vi "MyrioProject.vi"() -> ()   [LabVIEW 2018]
doc: "The myRIO Project template acquires acceleration data from the onboard accelerometer and displays the changes of acceleration values in a waveform chart."
uses:
  <vilib>/myRIO/Common/Instrument Driver Framework/myRIO v1.0/Encoder/typedefs/Encoder Signal Mode.ctl
  <vilib>/Platform/TimedLoop/XDataNode/timing_clust.ctl
  <vilib>/Platform/TimedLoop/XDataNode/nitl_modes.ctl
  <vilib>/Platform/TimedLoop/XDataNode/wakeup.ctl
  <vilib>/Analysis/Matrix/Datatypes/RealMatrix.ctl
  <vilib>/myRIO/Instrument Drivers/Onboard IO/PWM/typedefs/PWM Reference.ctl
  <vilib>/myRIO/Common/Instrument Driver Framework/Utilities/typedefs/myRIO Generic Hardware Reference.ctl
  <vilib>/myRIO/Common/Instrument Driver Framework/Utilities/typedefs/Hardware Version Enum.ctl
  <vilib>/myRIO/Common/Instrument Driver Framework/Utilities/typedefs/myRIO v1.0 Reference.ctl
  <vilib>/myRIO/Common/Instrument Driver Framework/Utilities/typedefs/Generic FPGA Reference.ctl
  <vilib>/myRIO/Common/Instrument Driver Framework/myRIO v1.0/PWM/typedefs/PWM Channels Enum.ctl
  <vilib>/myRIO/Instrument Drivers/Onboard IO/PWM/typedefs/PWM Configuration.ctl
  <vilib>/userdefined/High Color/nirio_resource_hc.ctl
  <vilib>/myRIO/Common/Instrument Driver Framework/myRIO v1.0/Encoder/typedefs/Encoder Configuration v1.0.ctl
  <vilib>/myRIO/Instrument Drivers/Onboard IO/Encoder/typedefs/Encoder Reference.ctl
  <vilib>/myRIO/Common/Instrument Driver Framework/myRIO v1.0/Encoder/typedefs/Encoder Channels Enum.ctl
  <vilib>/myRIO/Instrument Drivers/Onboard IO/DIO/typedefs/DIO Reference.ctl
  <vilib>/myRIO/Common/Instrument Driver Framework/myRIO v1.0/DIO/typedefs/DIO Channels List.ctl
  <vilib>/myRIO/Common/Instrument Driver Framework/myRIO v1.0/DIO/typedefs/DIO Channels Enum.ctl
  <vilib>/myRIO/Instrument Drivers/Onboard IO/AI/typedefs/AI Reference.ctl
  <vilib>/myRIO/Common/Instrument Driver Framework/myRIO v1.0/AI/typedefs/AI Channels List.ctl
  <vilib>/myRIO/Common/Instrument Driver Framework/myRIO v1.0/AI/typedefs/AI Channels Enum.ctl
  <vilib>/myRIO/Common/Instrument Driver Framework/Utilities/typedefs/Analog Scaling Constants List.ctl
  <vilib>/myRIO/Common/Instrument Driver Framework/Utilities/typedefs/Analog Scaling Constants.ctl
  <vilib>/myRIO/Common/Instrument Driver Framework/myRIO v1.0/PWM/vis/myRIO v1.1 Open PWM.vi
  <vilib>/myRIO/Common/Instrument Driver Framework/myRIO v1.0/Encoder/vis/myRIO v1.1 Open Encoder.vi
  <vilib>/myRIO/Common/Instrument Driver Framework/Utilities/vis/Is FPGA Ref Available.vi
  <vilib>/myRIO/Common/Instrument Driver Framework/myRIO v1.0/AI/vis/myRIO v1.1 Open AI.vi
  <vilib>/myRIO/Common/Instrument Driver Framework/myRIO v1.0/DIO/vis/myRIO v1.1 Open DIO.vi
  <vilib>/myRIO/Instrument Drivers/Onboard IO/PWM/vis/Set Duty Cycle and Frequency.vi
  <vilib>/myRIO/Instrument Drivers/Onboard IO/DIO/vis/Write.vi
  <vilib>/myRIO/Common/Instrument Driver Framework/Utilities/vis/Validate Channels.vi
  <vilib>/myRIO/Common/Instrument Driver Framework/myRIO v1.0/PWM/vis/myRIO v1.0 Reserve PWM.vi
  <vilib>/myRIO/Common/Instrument Driver Framework/myRIO v1.0/Encoder/vis/myRIO v1.0 Reserve Encoder.vi
  <vilib>/myRIO/Common/Instrument Driver Framework/myRIO v1.0/AI/vis/myRIO v1.0 Reserve AI.vi
  <vilib>/myRIO/Common/Instrument Driver Framework/myRIO v1.0/DIO/vis/myRIO v1.0 Reserve DIO.vi
  <vilib>/myRIO/Common/Instrument Driver Framework/myRIO v1.0/Encoder/vis/myRIO v1.0 Close Encoder.vi
  <vilib>/myRIO/Common/Instrument Driver Framework/myRIO v1.0/PWM/vis/myRIO v1.0 Close PWM.vi
  <vilib>/myRIO/Common/Instrument Driver Framework/myRIO v1.0/PWM/vis/myRIO v1.0 Build MUX Configuration PWM.vi
  <vilib>/myRIO/Common/Instrument Driver Framework/myRIO v1.0/Resource Manager/vis/myRIO v1.0 Reserve Channel List.vi
  <vilib>/myRIO/Common/Instrument Driver Framework/myRIO v1.0/Encoder/vis/myRIO v1.0 Build MUX Configuration Encoder.vi
  <vilib>/myRIO/Common/Instrument Driver Framework/myRIO v1.0/AI/vis/myRIO v1.0 Build MUX Configuration AI.vi
  <vilib>/myRIO/Common/Instrument Driver Framework/myRIO v1.0/DIO/vis/myRIO v1.0 Build MUX Configuration DIO.vi
  <vilib>/myRIO/Common/Instrument Driver Framework/myRIO v1.0/Encoder/vis/myRIO v1.0 Unreserve Encoder.vi
  <vilib>/myRIO/Common/Instrument Driver Framework/myRIO v1.0/PWM/vis/myRIO v1.0 Unreserve PWM.vi
  <vilib>/myRIO/Common/Instrument Driver Framework/myRIO v1.0/Resource Manager/vis/myRIO v1.0 Create Configuration List.vi
  <vilib>/myRIO/Common/Instrument Driver Framework/myRIO v1.0/Resource Manager/vis/myRIO v1.0 Reserve Channel.vi
  <vilib>/myRIO/Common/Instrument Driver Framework/myRIO v1.0/Resource Manager/vis/myRIO v1.0 Unreserve Channel.vi
  <vilib>/myRIO/Common/Instrument Driver Framework/myRIO v1.0/Resource Manager/vis/myRIO v1.0 Unreserve Channel List.vi
  <vilib>/myRIO/Common/Instrument Driver Framework/myRIO v1.0/Resource Manager/vis/myRIO v1.0 Build Mutex Name.vi
  <vilib>/Utility/VariantDataType/GetNumericInfo.vi
  <vilib>/Utility/error.llb/Error Cluster From Error Code.vi
  <vilib>/myRIO/Common/Instrument Driver Framework/myRIO v1.0/myRIO v1.1 Open.vi
  <vilib>/myRIO/Common/Instrument Driver Framework/Utilities/vis/IO Manager.vi
  <vilib>/myRIO/Common/Instrument Driver Framework/Utilities/vis/Configuration Manager.vi
  <vilib>/myRIO/Common/Instrument Driver Framework/myRIO v1.0/Resource Manager/vis/myRIO v1.0 Configure IO.vi
  <vilib>/myRIO/Common/Instrument Driver Framework/myRIO v1.0/myRIO v1.0 Close.vi
  <vilib>/myRIO/Common/Instrument Driver Framework/myRIO v1.0/PWM/vis/myRIO v1.0 Write PWM.vi
  <vilib>/myRIO/Common/Instrument Driver Framework/myRIO v1.0/Encoder/vis/myRIO v1.0 Configure Encoder.vi
  <vilib>/myRIO/Common/Instrument Driver Framework/myRIO v1.0/Encoder/vis/myRIO v1.0 Enable Encoder.vi
  <vilib>/myRIO/Common/Instrument Driver Framework/myRIO v1.0/DIO/vis/myRIO v1.0 Read DIO.vi
  <vilib>/myRIO/Common/Instrument Driver Framework/myRIO v1.0/AI/vis/myRIO v1.0 Get Scaling Constants AI.vi
  <vilib>/myRIO/Common/Instrument Driver Framework/myRIO v1.0/AI/vis/myRIO v1.0 Read AI.vi
  <vilib>/myRIO/Common/Instrument Driver Framework/myRIO v1.0/Encoder/vis/myRIO v1.0 Read Encoder.vi
  <vilib>/myRIO/Common/Instrument Driver Framework/myRIO v1.0/DIO/vis/myRIO v1.0 Write DIO.vi
  <vilib>/myRIO/Common/Instrument Driver Framework/myRIO v1.0/Encoder/vis/myRIO v1.0 Shutdown Encoder.vi
  <vilib>/myRIO/Common/Instrument Driver Framework/myRIO v1.0/PWM/vis/myRIO v1.0 Shutdown PWM.vi
  <vilib>/platform/TimedLoop/XDataNode/XDataNode.xnode
  <vilib>/myRIO/Instrument Drivers/Onboard IO/PWM/vis/myRIO PWM Open.xnode
  <vilib>/myRIO/Instrument Drivers/Onboard IO/Encoder/vis/myRIO Encoder Open.xnode
  <vilib>/myRIO/Express VI/Onboard IO/PWM/PWM Express VI.xnode
  <vilib>/myRIO/Express VI/Onboard Devices/Button/Button Express VI.xnode
  <vilib>/myRIO/Instrument Drivers/Onboard IO/DIO/vis/myRIO DIO Open.xnode
  <vilib>/myRIO/Express VI/Onboard IO/AI/AI Express VI.xnode
  <vilib>/myRIO/Instrument Drivers/Onboard IO/AI/vis/myRIO AI Open.xnode
  <vilib>/myRIO/Express VI/Onboard IO/DO/DO Express VI.xnode
  <vilib>/myRIO/Instrument Drivers/Onboard IO/Encoder/Encoder.lvlib
  <vilib>/myRIO/Instrument Drivers/Onboard IO/PWM/PWM.lvlib
  <vilib>/myRIO/Instrument Drivers/Onboard IO/DIO/DIO.lvlib
  <vilib>/myRIO/Instrument Drivers/Onboard IO/AI/AI.lvlib
  <vilib>/Platform/TimedLoop/XDataNode/XDNodeRunTimeDep.lvlib
  <vilib>/Analysis/Matrix/NI_Matrix.lvlib
panel:
  in  "Start":bool
  in  "Stop Button":bool
  out "element":dbl
  out "element 2":dbl
  in  "manual":bool
  out "Numeric Control":dbl
  out "data":dbl
  out "sensor2 (A/AI2 (Pin 7))":dbl
  out "sensor1":dbl
  out "stallRojo (A/AI0 (Pin 3))":dbl
  out "stallBlanco (A/AI1 (Pin 5))":dbl
  out "subarray 2":dbl[][](array[numeric])
  out "subarray":dbl[][](array[numeric])
  out "vectores":dbl[][][](array[numeric])
  in  "saturacion":dbl=0.3
  in  "Duty Cycle 2":dbl(slide)=0.5 scale=0.05..0.1
  in  "Duty Cycle":dbl(slide)=0.5 scale=0.05..0.1
  in  "Reset Counter 2":bool
  in  "Reset Counter":bool
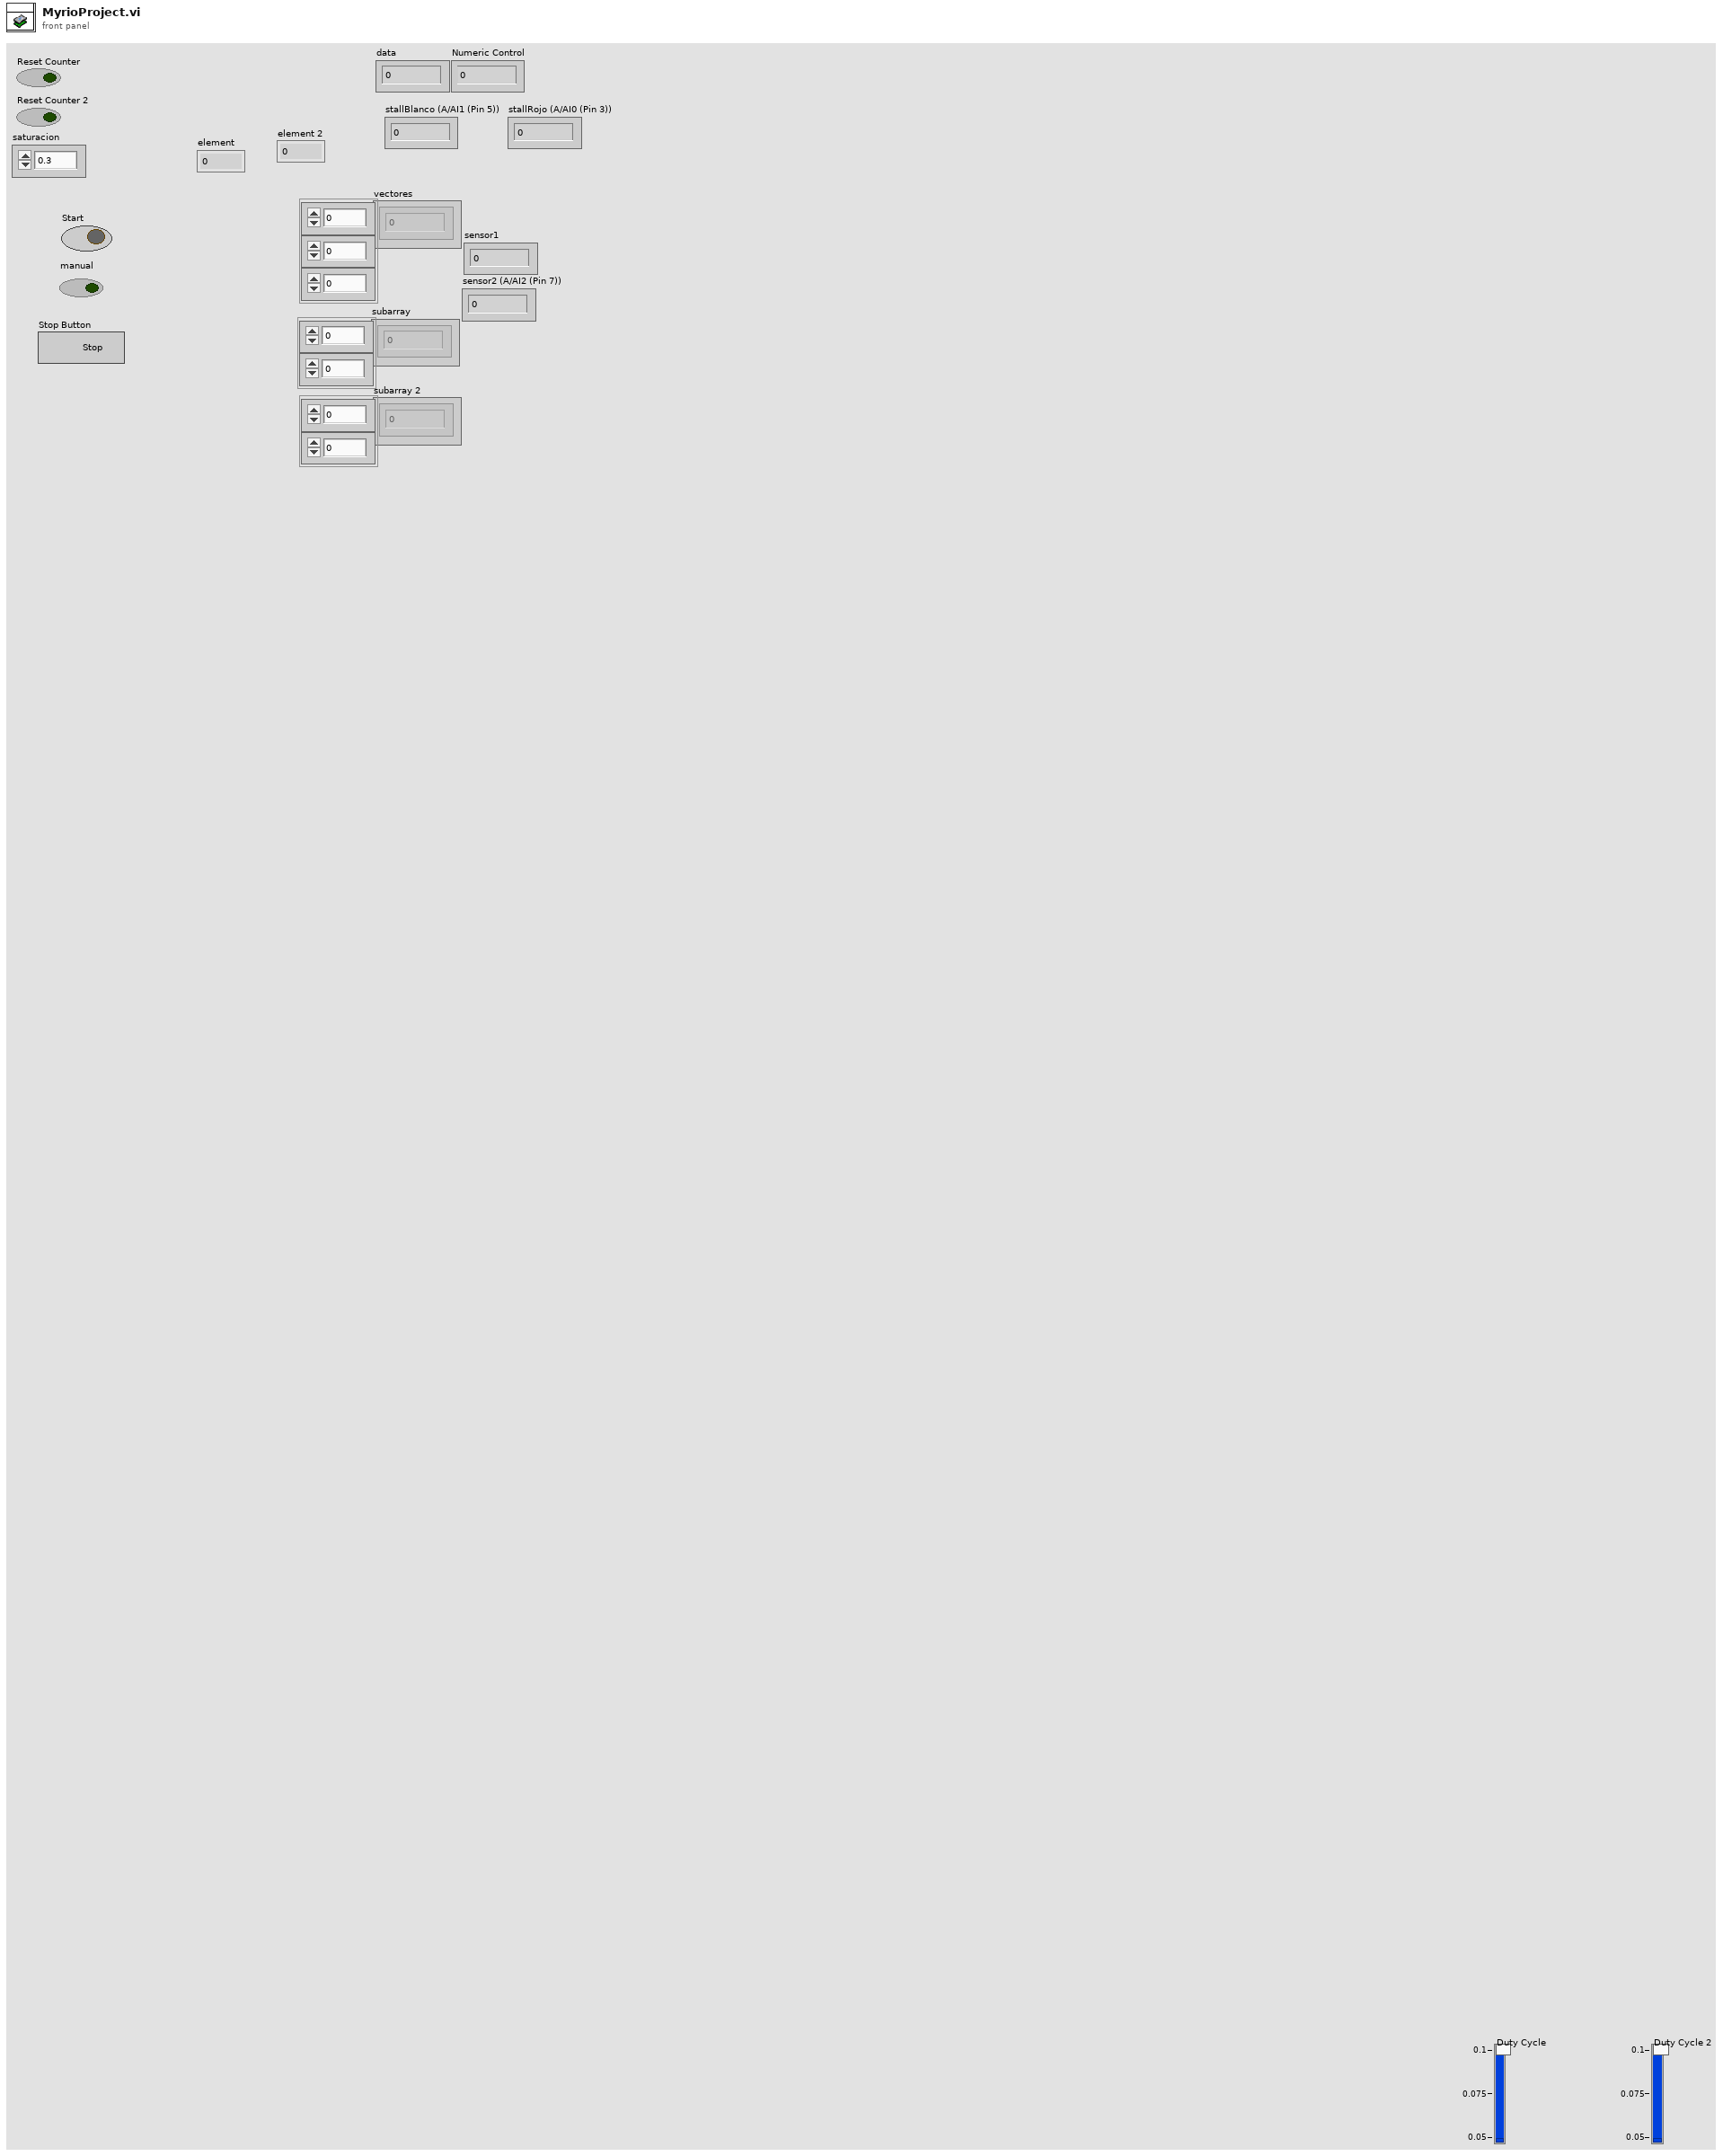
[diagram p1: front panel]
types:
  T1 = typedef "NI_Matrix.lvlib/RealMatrix.ctl" = dbl[][]
  T2 = enum16{"normal", "grande-Sensor", "grande home", "peque-sensor", "peque- home", "peque-reset"}
  T3 = typedef "Encoder Signal Mode.ctl" = enum16{"Quadrature phase signal", "Step and direction signal"}
  T4 = typedef "PWM.lvlib/PWM Reference.ctl" = cluster{"myRIO Reference":T5, "PWM Channels Enum":T9, "PWM Configuration":T10}
  T5 = typedef "myRIO Generic Hardware Reference.ctl" = cluster{"myRIO Model":T6, "myRIO Hardware Reference":T7}
  T6 = typedef "Hardware Version Enum.ctl" = enum16{"Unknown", "myRIO-1900", "myRIO-1950", "roboRIO", "NI ELVIS RIO CM", "ELVIS III"}
  T7 = typedef "myRIO v1.0 Reference.ctl" = cluster{"Generic FPGA Reference":T8, "Allow multiple opens":bool}
  T8 = typedef "Generic FPGA Reference.ctl" = refnum<k20>
  T9 = typedef "PWM Channels Enum.ctl" = enum16{"Not Connected", "C/PWM0", "C/PWM1", "A/PWM0", "A/PWM1", "A/PWM2", "A/PWM3", "A/PWM4", "A/PWM5", "A/PWM6", "A/PWM7", "A/PWM8", "A/PWM9", "A/PWM10", "A/PWM11", "A/PWM12", "A/PWM13", "A/PWM14", "A/PWM15", "A/PWM16", "A/PWM17", "A/PWM18", "A/PWM19", "B/PWM0", "B/PWM1", "B/PWM2", "B/PWM3", "B/PWM4", "B/PWM5", "B/PWM6", "B/PWM7", "B/PWM8", "B/PWM9", "B/PWM10", "B/PWM11", "B/PWM12", "B/PWM13", "B/PWM14", "B/PWM15", "B/PWM16", "B/PWM17", "B/PWM18", "B/PWM19", "PWM/PWM0", "PWM/PWM1", "PWM/PWM2", "PWM/PWM3", "PWM/PWM4", "PWM/PWM5", "PWM/PWM6", "PWM/PWM7", "PWM/PWM8", "PWM/PWM9"}
  T10 = typedef "PWM.lvlib/PWM Configuration.ctl" = cluster{"Frequency":dbl, "Duty Cycle":dbl}
  T11 = typedef "Encoder.lvlib/Encoder Reference.ctl" = cluster{"myRIO Reference":T5, "Encoder Channels Enum":T12}
  T12 = typedef "Encoder Channels Enum.ctl" = enum16{"Not Connected", "C/ENC0", "C/ENC1", "A/ENC", "A/ENC0", "A/ENC1", "A/ENC2", "A/ENC3", "A/ENC4", "A/ENC5", "A/ENC6", "A/ENC7", "A/ENC8", "A/ENC9", "B/ENC", "B/ENC0", "B/ENC1", "B/ENC2", "B/ENC3", "B/ENC4", "B/ENC5", "B/ENC6", "B/ENC7", "B/ENC8", "B/ENC9", "DIO/ENC0", "DIO/ENC1", "DIO/ENC2", "DIO/ENC3", "DIO/ENC4"}
  T13 = cluster{"Double":dbl, "dbl Scaled Value":dbl, "Output":dbl, "seconds since 1Jan1904":timestamp, dbl, dbl, dbl}
  T14 = typedef "XDNodeRunTimeDep.lvlib/timing_clust.ctl" = cluster{"Expected End [f-1]":u64, "Actual End [f-1]":u64, "Finished Late? [f-1]":bool, "Expected End [i-1]":u64, "Actual End [i-1]":u64, "Finished Late? [i-1]":bool, "Expected Start [i]":u64, "Actual Start [i]":u64, "Expected Start [f]":u64, "Actual Start [f]":u64, "Source Name":string, "Structure Name":string, "Period":i64, "Deadline":i64, "Offset":i64, "Start":i64, "Priority":i32, "Timeout":i32, "Mode":T15, "Wakeup Reason":T16, "Error":errorcluster, "Source Type":string, "Secondary Source Type":string, "Global End Time":u64, "Global Start Time":u64, "Frame Duration":u64, "Iteration Duration":u64, "Assigned CPU":i32, "I/O Scan Engine Mode":u32}
  T15 = typedef "XDNodeRunTimeDep.lvlib/nitl_modes.ctl" = enum32{"No Change", "Process missed periods, maintain original phase", "Discard missed periods, maintain original phase", "Process missed periods, ignore original phase", "Discard missed periods, ignore original phase"}
  T16 = typedef "XDNodeRunTimeDep.lvlib/wakeup.ctl" = enum32{"Normal", "Aborted", "Asynchronous wakeup", "Timing source error", "Timed loop error", "Timeout"}
  T17 = typedef "nirio_resource_hc.ctl" = tag
  T18 = typedef "AI.lvlib/AI Reference.ctl" = cluster{"myRIO Reference":T5, "AI Channels List":T19, "AI Scaling Constants List":T21}
  T19 = typedef "AI Channels List.ctl" = T20[]
  T20 = typedef "AI Channels Enum.ctl" = enum16{"Not Connected", "AudioIn/Left", "AudioIn/Right", "C/AI0", "C/AI1", "A/AI0", "A/AI1", "A/AI2", "A/AI3", "A/AI4", "A/AI5", "A/AI6", "A/AI7", "B/AI0", "B/AI1", "B/AI2", "B/AI3", "B/AI4", "B/AI5", "B/AI6", "B/AI7", "AI/AI0", "AI/AI1", "AI/AI2", "AI/AI3", "A/AI0 (DIFF)", "A/AI1 (DIFF)", "A/AI2 (DIFF)", "A/AI3 (DIFF)", "B/AI0 (DIFF)", "B/AI1 (DIFF)", "B/AI2 (DIFF)", "B/AI3 (DIFF)"}
  T21 = typedef "Analog Scaling Constants List.ctl" = T22[]
  T22 = typedef "Analog Scaling Constants.ctl" = cluster{"LSB Weight (Volts)":dbl, "Offset (Volts)":dbl, "Signed?":bool}
  T23 = typedef "DIO.lvlib/DIO Reference.ctl" = cluster{"myRIO Reference":T5, "DIO Channels List":T24}
  T24 = typedef "DIO Channels List.ctl" = T25[]
  T25 = typedef "DIO Channels Enum.ctl" = enum16{"Not Connected", "C/DIO0", "C/DIO1", "C/DIO2", "C/DIO3", "C/DIO4", "C/DIO5", "C/DIO6", "C/DIO7", "A/DIO0", "A/DIO1", "A/DIO2", "A/DIO3", "A/DIO4", "A/DIO5", "A/DIO6", "A/DIO7", "A/DIO8", "A/DIO9", "A/DIO10", "A/DIO11", "A/DIO12", "A/DIO13", "A/DIO14", "A/DIO15", "A/DIO16", "A/DIO17", "A/DIO18", "A/DIO19", "B/DIO0", "B/DIO1", "B/DIO2", "B/DIO3", "B/DIO4", "B/DIO5", "B/DIO6", "B/DIO7", "B/DIO8", "B/DIO9", "B/DIO10", "B/DIO11", "B/DIO12", "B/DIO13", "B/DIO14", "B/DIO15", "B/DIO16", "B/DIO17", "B/DIO18", "B/DIO19", "LED0", "LED1", "LED2", "LED3", "Button0", "DIO/DIO0", "DIO/DIO1", "DIO/DIO2", "DIO/DIO3", "DIO/DIO4", "DIO/DIO5", "DIO/DIO6", "DIO/DIO7", "DIO/DIO8", "DIO/DIO9", "SPI/CS0", "SPI/CS1", "SPI/CS2", "SPI/CS3", "LED RADIO (Green)", "LED RADIO (Red)", "LED COMM (Green)", "LED COMM (Red)", "LED MODE (Green)", "LED MODE (Red)"}
  T26 = cluster{dbl, dbl, "Counter Value":i32, "seconds since 1Jan1904":timestamp, dbl, dbl, "Counter Value":i32}
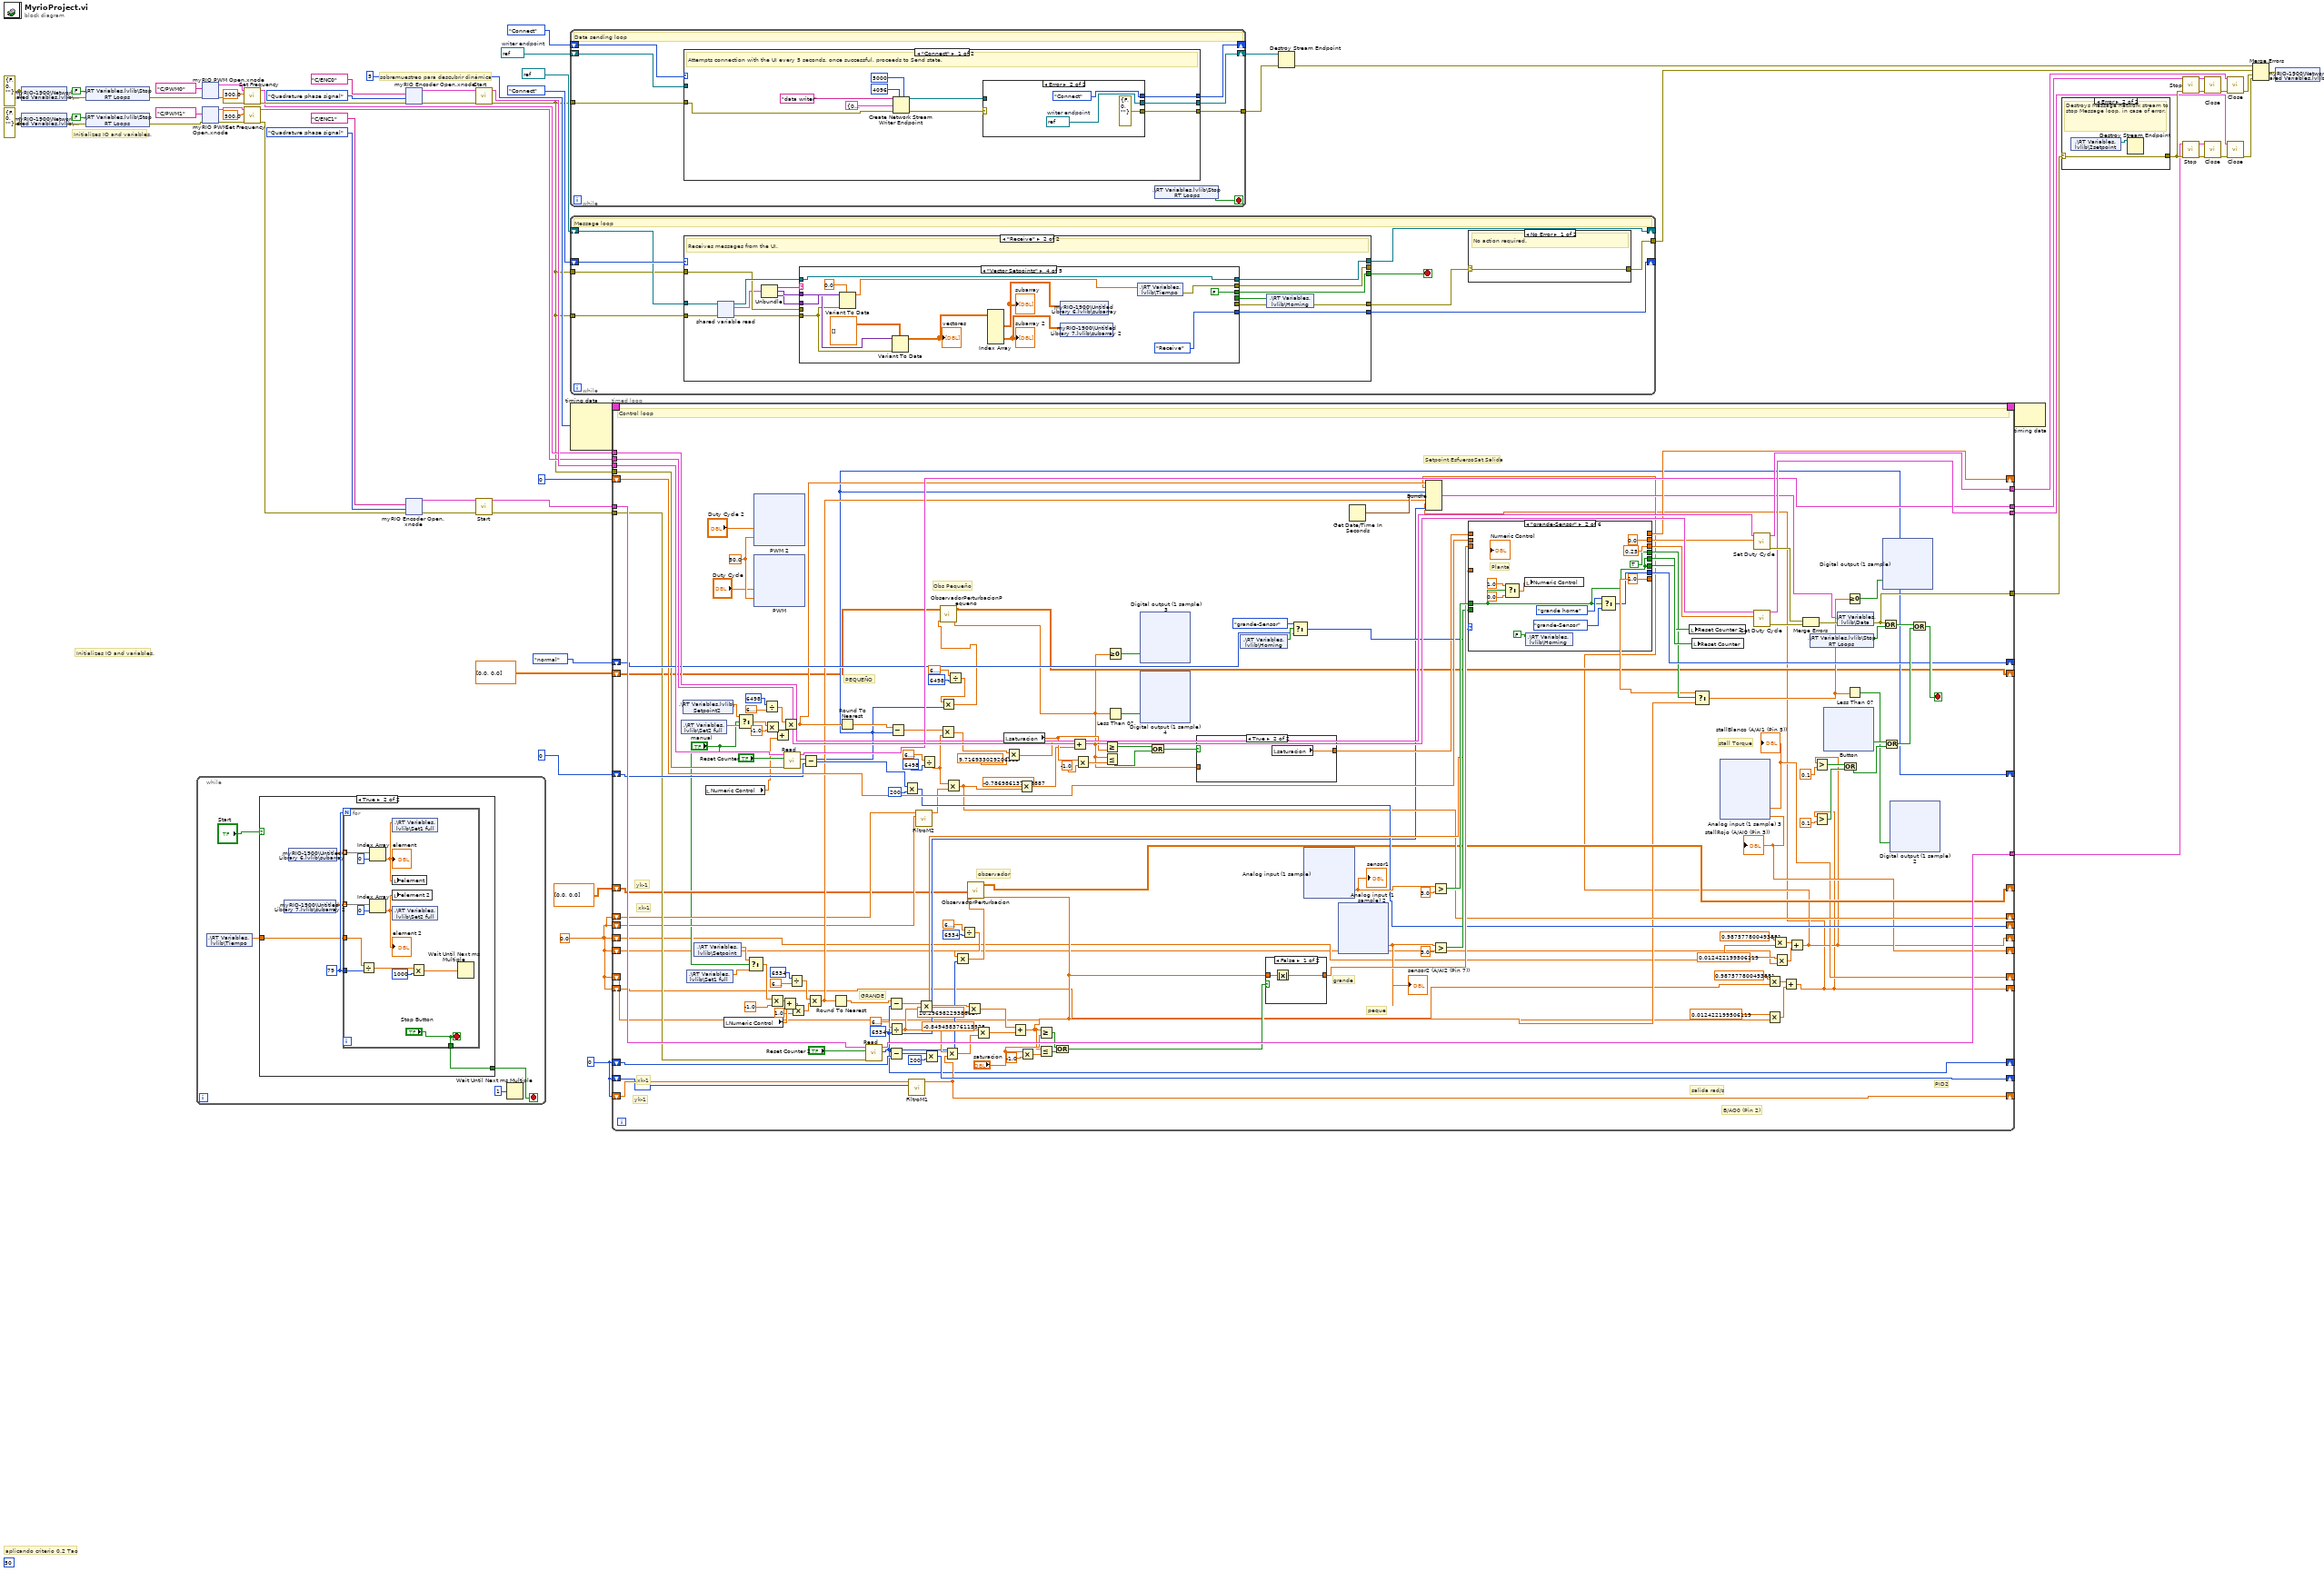
[diagram p0: block diagram]
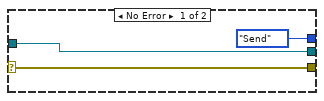
[diagram p4: hidden frame]
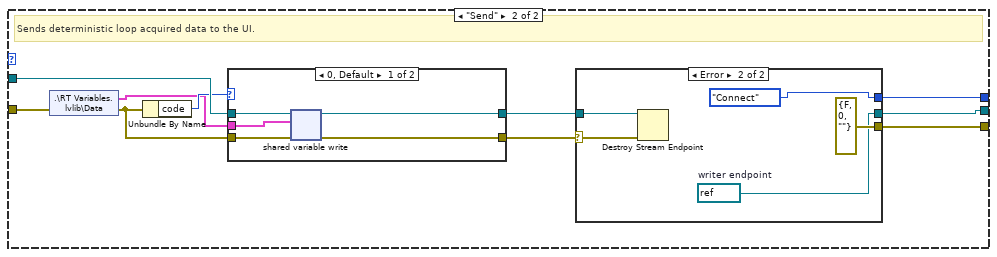
[diagram p5: hidden frame]
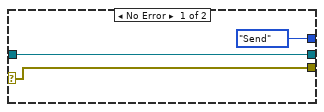
[diagram p6: hidden frame]
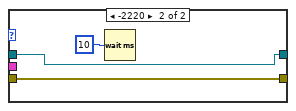
[diagram p7: hidden frame]
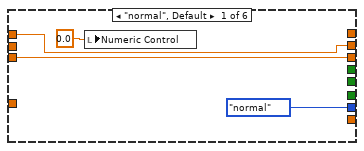
[diagram p8: hidden frame]
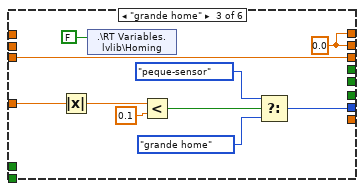
[diagram p9: hidden frame]
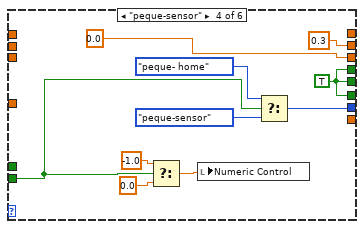
[diagram p10: hidden frame]
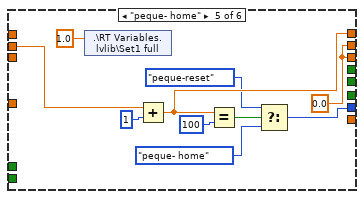
[diagram p11: hidden frame]
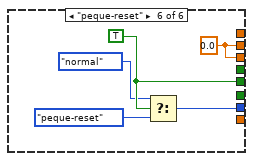
[diagram p12: hidden frame]
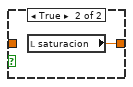
[diagram p13: hidden frame]
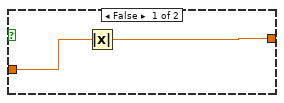
[diagram p14: hidden frame]
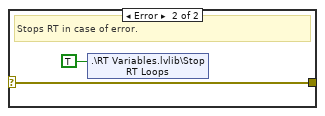
[diagram p15: hidden frame]
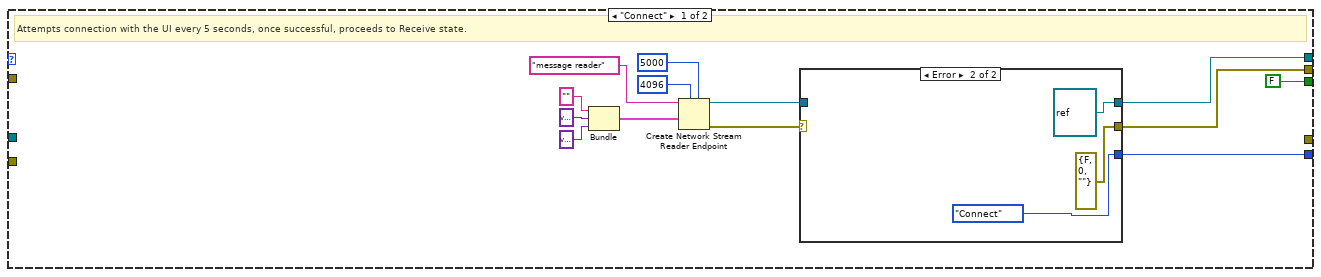
[diagram p16: hidden frame]
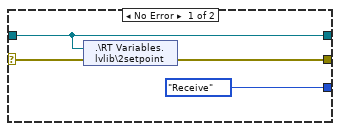
[diagram p17: hidden frame]
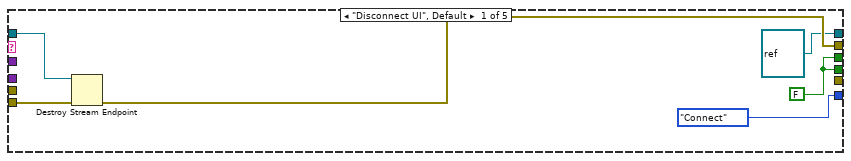
[diagram p18: hidden frame]
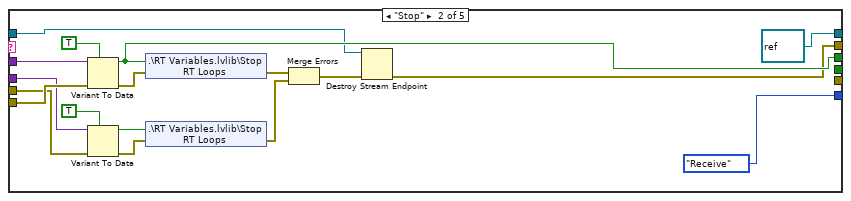
[diagram p19: hidden frame]
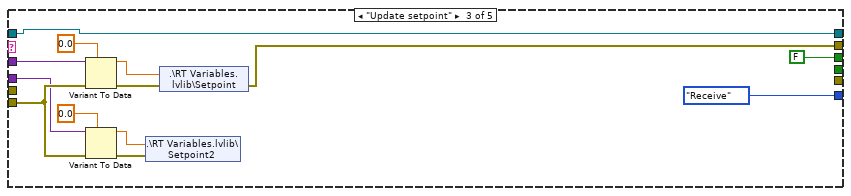
[diagram p20: hidden frame]
diagram:
  w1 = 0.0
  w2 = 0 ("Counter Value")
  (unwired) 50
  w19 = refnum<k21> refnum  # writer endpoint
  w32 = errorcluster {"status"=FALSE, "code"=0, "source"=""} ("error IO")
  w54 = errorcluster {"status"=FALSE, "code"=0, "source"=""} ("error IO")
  # "aplicando criterio 0.2 Tao"
  # "sobremuestreo para descubrir dinámica"
  # "Initializes IO and variables."
  # "Initializes IO and variables."
  n1 = shared-variable "myRIO-1900\\Network Shared Variables.lvlib\\error IO"(w54, error in=w54) -> (error out=w55:errorcluster)
  n2 = shared-variable "myRIO-1900\\Network Shared Variables.lvlib\\error IO"(w32, error in=w32) -> (error out=w33:errorcluster)
  n3 = shared-variable ".\\RT Variables.lvlib\\Stop RT Loops"(FALSE ("Stop RT Loops"), error in=w55) -> (error out=w42:errorcluster)
  n4 = shared-variable ".\\RT Variables.lvlib\\Stop RT Loops"(FALSE ("Stop RT Loops"), error in=w33) -> (error out=w25:errorcluster)
  n5 = while {
    stop <- w66 stop-if-true
    n6 = shared-variable ".\\RT Variables.lvlib\\Tiempo"() -> (w68:dbl)  [unwired: 1 in, 1 out]
    n7 = case shown="True" "Start" {
      tunnel: w68 -> [_ w71]
      tunnel: [_ w70] -> w66
      frame False {
      }
      frame True {
        w74 = 79
        n8 = shared-variable "myRIO-1900\\Untitled Library 7.lvlib\\subarray 2"() -> (w72:dbl[][])  [unwired: 1 in, 1 out]
        n9 = shared-variable "myRIO-1900\\Untitled Library 6.lvlib\\subarray"() -> (w73:dbl[][])  [unwired: 1 in, 1 out]
        n10 = for {
          N: w74 -> [_]
          tunnel: w74 -> [w84]
          tunnel: w73 -> [w83] mode=indexing
          tunnel: w72 -> [w80] mode=indexing
          tunnel: w71 -> [w76]
          tunnel: ["Stop Button"] -> w70
          stop <- "Stop Button" stop-if-true
          n11 = Divide(x=w76, y=w84) -> (x/y=w86:dbl)
          n12 = Index Array(array=w83, index=0) -> (element=w78:dbl)
          "element" <- w78
          n13 = Index Array(array=w80, index=0) -> (element=w77:dbl)
          "element 2" <- w77
          n14 = shared-variable ".\\RT Variables.lvlib\\Set1 full"(w78) -> ()  [unwired: 1 in, 1 out]
          n15 = local write "element"(w78) -> ()
          n16 = local write "element 2"(w77) -> ()
          n17 = shared-variable ".\\RT Variables.lvlib\\Set2 full"(w77) -> ()  [unwired: 1 in, 1 out]
          n18 = Multiply(x=w86, y=1000) -> (x*y=w79:dbl)
          n19 = Wait Until Next ms Multiple(millisecond multiple=w79) -> ()  [unwired: 1 out]
        }
      }
    }
    n20 = Wait Until Next ms Multiple(millisecond multiple=u32 1) -> ()  [unwired: 1 out]
  }
  n21 = xnode "myRIO PWM Open.xnode"("error in (no error)"=w42, "Channel Name"=tag "C/PWM0") -> ("error out"=w44:errorcluster, "PWM Ref Out"=w43:T4)  [unwired: 1 in]
  n22 = xnode "myRIO PWM Open.xnode"("error in (no error)"=w25, "Channel Name"=tag "C/PWM1") -> ("error out"=w27:errorcluster, "PWM Ref Out"=w26:T4)  [unwired: 1 in]
  n23 = call <vilib>:"Set Frequency.vi"("error in (no error)"=w44, "Frequency [Hz]"=500.0, "PWM Ref In"=w43) -> ("error out"=w41:errorcluster, "PWM Ref Out"=w38:T4)  [unwired: 6 in]
  n24 = call <vilib>:"Set Frequency.vi"("error in (no error)"=w27, "Frequency [Hz]"=500.0, "PWM Ref In"=w26) -> ("error out"=w24:errorcluster, "PWM Ref Out"=w20:T4)  [unwired: 6 in]
  n25 = xnode "myRIO Encoder Open.xnode"("error in (no error)"=w41, "Channel Name"=tag "C/ENC0", "Encoder Signal Mode"=Encoder_Signal_Mode."Quadrature phase signal") -> ("error out"=w51:errorcluster, "Encoder Ref Out"=w50:T11)  [unwired: 2 in]
  n26 = xnode "myRIO Encoder Open.xnode"("error in (no error)"=w24, "Channel Name"=tag "C/ENC1", "Encoder Signal Mode"=Encoder_Signal_Mode."Quadrature phase signal") -> ("error out"=w30:errorcluster, "Encoder Ref Out"=w29:T11)  [unwired: 2 in]
  n27 = call <vilib>:"Start.vi"("error in (no error)"=w51, "Encoder Ref In"=w50) -> ("error out"=w9:errorcluster, "Encoder Ref Out"=w48:T11)  [unwired: 8 in]
  n28 = call <vilib>:"Start.vi"("error in (no error)"=w30, "Encoder Ref In"=w29) -> ("error out"=w8:errorcluster, "Encoder Ref Out"=w21:T11)  [unwired: 8 in]
  n29 = while {
    shift-right: [w91] -> w60
    shift-left: w19 -> [w89]
    tunnel: [w90] -> w61
    tunnel: w9 -> [w88]
    shift-right: [w87] -> _
    shift-left: enum16{"Connect", "Send"}."Connect" ("Message states") -> [w92]
    stop <- w93 stop-if-true
    # "Data sending loop"
    n30 = case shown="\"Connect\"" w92 {
      tunnel: [w97 w112] -> w90
      tunnel: [w95 w110] -> w91
      tunnel: [w101 w113] -> w87
      tunnel: w89 -> [_ w119]
      tunnel: w88 -> [w98 w118]
      frame "Connect" {
        # "Attempts connection with the UI every 5 seconds, once successful, proceeds to Send state."
        n31 = Create Network Stream Writer Endpoint(5:5000 ("timeout in ms (-1)"), 7:4096 ("writer buffer size"), 8:w98, 9:T13 {"Double"=0.0, "dbl Scaled Value"=0.0, "Output"=0.0, "seconds since 1Jan1904"=timestamp(0 s since 1904-01-01), 0.0, 0.0, 0.0} ("Data"), 11:"data writer" ("writer name")) -> (0:w99:errorcluster, 3:w96:refnum<k21>)  [unwired: 2 in]
        n32 = case shown="Error" w99 {
          selector: w99 -> [w104 _]
          tunnel: [enum16{"Connect", "Send"}."Send" ("Message states") enum16{"Connect", "Send"}."Connect" ("Message states")] -> w101
          tunnel: [w104 errorcluster {"status"=FALSE, "code"=0, "source"=""} ("error IO")] -> w97
          tunnel: w96 -> [w106 _]
          tunnel: [w106 w107] -> w95
          frame No Error {
          }
          frame Error {
            w107 = refnum<k21> refnum  # writer endpoint
          }
        }
      }
      frame "Send" {
        # "Sends deterministic loop acquired data to the UI."
        n33 = shared-variable ".\\RT Variables.lvlib\\Data"(error in=w118) -> (w115:T13, error out=w117:errorcluster)
        n34 = Unbundle By Name(w117) -> ("code"=w116:i32)
        n35 = case shown="0, Default" w116 {
          tunnel: [w132 w134] -> w114
          tunnel: [w131 w133] -> w111
          tunnel: w119 -> [w130 w133]
          tunnel: w117 -> [w129 w134]
          tunnel: w115 -> [w128 _]
          frame 0, Default {
            n36 = shared-variable-write(w130, w129, w128) -> (w131:refnum<k21>, w132:errorcluster)  [unwired: 1 in, 1 out]
          }
          frame -2220 {
            n37 = Wait (ms)(milliseconds to wait=u32 10) -> ()  [unwired: 1 out]
          }
        }
        n38 = case shown="Error" w114 {
          selector: w114 -> [w122 w126]
          tunnel: [enum16{"Connect", "Send"}."Send" ("Message states") enum16{"Connect", "Send"}."Connect" ("Message states")] -> w113
          tunnel: [w122 errorcluster {"status"=FALSE, "code"=0, "source"=""} ("error IO")] -> w112
          tunnel: w111 -> [w120 w125]
          tunnel: [w120 w123] -> w110
          frame No Error {
          }
          frame Error {
            w123 = refnum<k21> refnum  # writer endpoint
            n39 = Destroy Stream Endpoint(8:w126, 11:w125) -> ()  [unwired: 1 out]
          }
        }
      }
    }
    n40 = shared-variable ".\\RT Variables.lvlib\\Stop RT Loops"() -> (w93:bool)  [unwired: 1 in, 1 out]
  }
  n41 = while {
    tunnel: [w139] -> w57
    shift-right: [w143] -> _
    shift-left: refnum<k21> refnum ("reader endpoint") -> [w141]
    shift-right: [w142] -> _
    shift-left: enum16{"Connect", "Receive"}."Connect" ("Message states") -> [w144]
    tunnel: w9 -> [w140]
    tunnel: w9 -> [w137]
    stop <- w138 stop-if-true
    # "Message loop"
    n42 = case shown="\"Receive\"" w144 {
      tunnel: [w151 w168] -> _
      tunnel: [w149 w180] -> w143
      tunnel: [w158 w177] -> w142
      tunnel: w141 -> [_ w176]
      tunnel: w140 -> [_ w179]
      tunnel: [FALSE ("Stop RT Loops") w178] -> w138
      tunnel: w137 -> [_ w173]
      tunnel: [_ w169] -> w136
      frame "Connect" {
        # "Attempts connection with the UI every 5 seconds, once successful, proceeds to Receive state."
        n43 = Bundle("", variant, variant) -> (w154:cluster{string, variant, variant})  [unwired: 1 in]
        n44 = Create Network Stream Reader Endpoint(5:5000 ("timeout in ms (-1)"), 7:4096 ("reader buffer size"), 9:w154, 11:"message reader" ("reader name")) -> (0:w153:errorcluster, 3:w148:refnum<k21>)  [unwired: 3 in]
        n45 = case shown="Error" w153 {
          selector: w153 -> [w163 _]
          tunnel: [enum16{"Connect", "Receive"}."Receive" ("Message states") enum16{"Connect", "Receive"}."Connect" ("Message states")] -> w158
          tunnel: [w162 errorcluster {"status"=FALSE, "code"=0, "source"=""} ("error IO")] -> w151
          tunnel: [w161 refnum<k21> refnum ("reader endpoint")] -> w149
          tunnel: w148 -> [w161 _]
          frame No Error {
            n46 = shared-variable ".\\RT Variables.lvlib\\2setpoint"(w161, error in=w163) -> (error out=w162:errorcluster)
          }
          frame Error {
          }
        }
      }
      frame "Receive" {
        # "Receives messages from the UI."
        n47 = shared-variable-read(w176, w179) -> (w175:refnum<k21>, w181:errorcluster, w172:cluster{string, variant, variant})  [unwired: 1 in, 1 out]
        n48 = Unbundle(w172) -> (w183:string, w182:variant, w174:variant)
        n49 = case shown="\"Vector Setpoints\"" w183 {
          tunnel: w182 -> [_ w204 w219 w225 w243]
          tunnel: w181 -> [w188 w206 w208 w224 w237]
          tunnel: [w187 w201 w215 w226 _] -> w168
          tunnel: [refnum<k21> refnum ("reader endpoint") refnum<k21> refnum ("reader endpoint") w214 w232 w241] -> w180
          tunnel: w175 -> [w186 w200 w214 w232 w241]
          tunnel: [w184 w203 FALSE ("Stop RT Loops") FALSE ("Stop RT Loops") FALSE ("Stop RT Loops")] -> w178
          tunnel: [enum16{"Connect", "Receive"}."Connect" ("Message states") enum16{"Connect", "Receive"}."Receive" ("Message states") enum16{"Connect", "Receive"}."Receive" ("Message states") enum16{"Connect", "Receive"}."Receive" ("Message states") enum16{"Connect", "Receive"}."Receive" ("Message states")] -> w177
          tunnel: w174 -> [_ w196 w207 w228 w236]
          tunnel: w173 -> [_ w195 _ _ _]
          tunnel: [w184 _ _ _ w234] -> w171
          tunnel: [_ _ _ _ w233] -> w170
          frame "Disconnect UI", Default {
            w184 = FALSE ("Stop RT Loops")
            n50 = Destroy Stream Endpoint(8:w188, 11:w186) -> (0:w187:errorcluster)
          }
          frame "Stop" {
            n51 = Variant To Data(error in=w206, type=TRUE ("Stop RT Loops"), Variant=w204) -> (data=w203:bool, error out=w205:errorcluster)
            n52 = Variant To Data(error in=w195, type=TRUE ("Stop RT Loops"), Variant=w196) -> (data=w193:bool, error out=w197:errorcluster)
            n53 = shared-variable ".\\RT Variables.lvlib\\Stop RT Loops"(w203, error in=w205) -> (error out=w191:errorcluster)
            n54 = shared-variable ".\\RT Variables.lvlib\\Stop RT Loops"(w193, error in=w197) -> (error out=w192:errorcluster)
            n55 = Merge Errors(w191, w192) -> (w190:errorcluster)
            n56 = Destroy Stream Endpoint(8:w190, 11:w200) -> (0:w201:errorcluster)
          }
          frame "Update setpoint" {
            n57 = Variant To Data(error in=w208, type=0.0, Variant=w219) -> (data=w217:dbl, error out=w216:errorcluster)
            n58 = Variant To Data(error in=w208, type=0.0, Variant=w207) -> (data=w210:dbl, error out=w209:errorcluster)
            n59 = shared-variable ".\\RT Variables.lvlib\\Setpoint2"(w210, error in=w209) -> ()  [unwired: 1 out]
            n60 = shared-variable ".\\RT Variables.lvlib\\Setpoint"(w217, error in=w216) -> (error out=w215:errorcluster)
          }
          frame "Vector Setpoints" {
            n61 = Variant To Data(error in=w224, type=0.0, Variant=w228) -> (data=w227:dbl)  [unwired: 1 out]
            n62 = Variant To Data(error in=w224, type=dbl[][][] [], Variant=w225) -> (data=w222:dbl[][][])  [unwired: 1 out]
            "vectores" <- w222
            n63 = Index Array(array=w222) -> (element #1=w221:dbl[][], element #2=w220:dbl[][])  [unwired: 6 in]
            "subarray" <- w221
            "subarray 2" <- w220
            n64 = shared-variable "myRIO-1900\\Untitled Library 6.lvlib\\subarray"(w221) -> ()  [unwired: 1 in, 1 out]
            n65 = shared-variable "myRIO-1900\\Untitled Library 7.lvlib\\subarray 2"(w220) -> ()  [unwired: 1 in, 1 out]
            n66 = shared-variable ".\\RT Variables.lvlib\\Tiempo"(w227) -> (error out=w226:errorcluster)  [unwired: 1 in]
          }
          frame "Homing" {
            n67 = Variant To Data(error in=w237, type=0.0, Variant=w236) -> (data=→"data":dbl)  [unwired: 1 out]
            n68 = Variant To Data(error in=w237, type=TRUE, Variant=w243) -> (data=w234:bool, error out=w233:errorcluster)
          }
        }
        n69 = shared-variable ".\\RT Variables.lvlib\\Homing"(w171, error in=w170) -> (error out=w169:errorcluster)
      }
    }
    n70 = case shown="No Error" w136 {
      selector: w136 -> [w145 w146]
      tunnel: [w145 w146] -> w139
      frame No Error {
        # "No action required."
      }
      frame Error {
        # "Stops RT in case of error."
        n71 = shared-variable ".\\RT Variables.lvlib\\Stop RT Loops"(TRUE ("Stop RT Loops")) -> ()  [unwired: 1 in, 1 out]
      }
    }
  }
  n72 = node-c288(i64 5 ("Period")) -> (w65:T14)  [unwired: 3 in]
  n73 = timed-loop {
    timing: w65 -> [_]
    timing-out: [_] -> w64
    tunnel: [w403] -> w53
    tunnel: w48 -> [w382]
    tunnel: [w381] -> w45
    tunnel: w38 -> [w370]
    tunnel: [w402] -> w37
    tunnel: w21 -> [w399]
    tunnel: w20 -> [w398]
    tunnel: [w394] -> w14
    tunnel: [w393] -> w13
    shift-right: [w368] -> _
    shift-left: T2."normal" ("Enum") -> [w367]
    shift-right: [w362] -> _
    shift-left: 0 -> [w361]
    shift-right: [w283] -> _
    shift-left: 0 -> [w354]
    tunnel: w8 -> [w349]
    tunnel: w9 -> [w348]
    shift-right: [w288] -> _
    shift-left: w2 -> [w303]
    shift-right: [w299] -> _
    shift-left: w2 -> [w297]
    shift-right: [w296] -> _
    shift-left: w2 -> [w298]
    shift-right: [w295] -> _
    shift-left: w1 -> [w294]
    shift-right: [w291] -> _
    shift-left: w1 -> [w293]
    shift-right: [w281] -> _
    shift-left: T1 [[0.0], [0.0]] ("A + B") -> [w282]
    shift-right: [w279] -> _
    shift-left: T1 [[0.0], [0.0]] ("A + B") -> [w278]
    shift-right: [w245] -> _
    shift-left: w1 -> [w255]
    shift-right: [w244] -> _
    shift-left: w1 -> [w250]
    shift-right: [w249] -> _
    shift-left: w1 -> [w248]
    shift-right: [w247] -> _
    shift-left: w1 -> [w246]
    stop <- w391 stop-if-true
    w351 = 50.0 ("Frequency [Hz]")
    # "Obs Pequeño"
    # "observador"
    # "yk-1"
    # "xk-1"
    # "yk-1"
    # "xk-1"
    # "PEQUEÑO"
    # "peque"
    # "grande"
    # "stall Torque"
    # "Setpoint,EsfuersoSat,Salida"
    # "PID2"
    # "GRANDE"
    # "salida rad/s"
    # "B/AO0 (Pin 2)"
    # "Control loop"
    n74 = shared-variable ".\\RT Variables.lvlib\\Set2 full"() -> (w270:dbl)  [unwired: 1 in, 1 out]
    n75 = shared-variable ".\\RT Variables.lvlib\\Setpoint2"() -> (w271:dbl)  [unwired: 1 in, 1 out]
    n76 = shared-variable ".\\RT Variables.lvlib\\Set1 full"() -> (w267:dbl)  [unwired: 1 in, 1 out]
    n77 = shared-variable ".\\RT Variables.lvlib\\Setpoint"() -> (w268:dbl)  [unwired: 1 in, 1 out]
    n78 = local read "Numeric Control"() -> (w264:dbl)
    n79 = local read "Numeric Control"() -> (w319:dbl)
    n80 = Select(t=w271, s="manual", f=w270) -> (s? t:f=w269:dbl)
    n81 = Select(t=w268, s="manual", f=w267) -> (s? t:f=w266:dbl)
    n82 = xnode "PWM 2"("Duty Cycle"="Duty Cycle 2", "Frequency [Hz]"=w351) -> ()  [unwired: 1 in, 1 out]
    n83 = xnode "PWM"("Duty Cycle"="Duty Cycle", "Frequency [Hz]"=w351) -> ()  [unwired: 1 in, 1 out]
    n84 = Divide(x=6498, y=6.283185307179586) -> (x/y=w343:dbl)
    n85 = Multiply(x=w269, y=-1.0) -> (x*y=w273:dbl)
    n86 = Multiply(x=w266, y=-1.0) -> (x*y=w318:dbl)
    n87 = Add(x=w273, y=w264) -> (x+y=w272:dbl)
    n88 = Add(x=w318, y=w319) -> (x+y=w276:dbl)
    n89 = Multiply(x=w343, y=w272) -> (x*y=w315:dbl)
    n90 = call <vilib>:"Read.vi"("error in (no error)"=w348, "Reset Counter"="Reset Counter", "Encoder Ref In"=w382) -> ("Counter Value"=w283:i32, "Encoder Ref Out"=w381:T11)  [unwired: 4 in, 3 out]
    n91 = Divide(x=6534, y=6.283185307179586) -> (x/y=w340:dbl)
    n92 = Multiply(x=w276, y=1.0) -> (x*y=w274:dbl)
    n93 = Subtract(x=w283, y=w354) -> (x-y=w329:i32)
    n94 = Multiply(x=w340, y=w274) -> (x*y=w311:dbl)
    n95 = Round To Nearest(number=w311) -> (nearest integer value=w385:dbl)
    n96 = Round To Nearest(number=w315) -> (nearest integer value=w380:dbl)
    n97 = call <vilib>:"Read.vi"("error in (no error)"=w349, "Reset Counter"="Reset Counter 2", "Encoder Ref In"=w399) -> ("Counter Value"=w288:i32, "Encoder Ref Out"=w394:T11)  [unwired: 4 in, 3 out]
    n98 = Subtract(x=w385, y=w288) -> (x-y=w261:dbl)
    n99 = Subtract(x=w288, y=w303) -> (x-y=w305:i32)
    n100 = Divide(x=6.283185307179586, y=6534) -> (x/y=w302:dbl)
    n101 = Subtract(x=w380, y=w283) -> (x-y=w260:dbl)
    n102 = Multiply(x=w329, y=200) -> (x*y=w295:i32)
    n103 = call "FiltroM1.vi"("Numeric 3"=w297, "Numeric in"=w298) -> ("Numeric out"=w296:dbl)  [unwired: 9 in]
    n104 = call "FiltroM2.vi"("Numeric 3"=w294, "Numeric in"=w293) -> ("Numeric out"=w292:dbl)  [unwired: 9 in]
    n105 = Multiply(x=w261, y=w302) -> (x*y=w308:dbl)
    n106 = Divide(x=6.283185307179586, y=6498) -> (x/y=w316:dbl)
    n107 = Multiply(x=w305, y=200) -> (x*y=w299:i32)
    n108 = Multiply(x=w260, y=w316) -> (x*y=w326:dbl)
    n109 = Multiply(x=w302, y=w296) -> (x*y=w304:dbl)
    n110 = Multiply(x=w316, y=w292) -> (x*y=w291:dbl)
    n111 = Divide(x=6.283185307179586, y=6498) -> (x/y=w284:dbl)
    n112 = Multiply(x=w284, y=w283) -> (x*y=w277:dbl)
    n113 = Divide(x=6.283185307179586, y=6534) -> (x/y=w287:dbl)
    n114 = Multiply(x=w287, y=w288) -> (x*y=w280:dbl)
    n115 = Multiply(x=w308, y=10.29698229388027) -> (x*y=w309:dbl)
    n116 = Multiply(x=-0.849458376115575, y=w304) -> (x*y=w301:dbl)
    n117 = local read "saturacion"() -> (w335:dbl)
    n118 = Multiply(x=w326, y=9.716933029206213) -> (x*y=w355:dbl)
    n119 = Add(x=w309, y=w301) -> (x+y=w262:dbl)
    n120 = call "ObservadorPerturbacion.vi"("entrada planta"=w262, "salida planta"=w280, "xk +1"=w282) -> ("xk"=w281:T1)  [unwired: 7 in, 1 out]
    n121 = Multiply(x=-0.786986137963887, y=w291) -> (x*y=w312:dbl)
    n122 = Multiply(x="saturacion", y=-1.0) -> (x*y=w334:dbl)
    n123 = Greater Or Equal?(x=w262, y="saturacion") -> (x >= y?=w388:bool)
    n124 = Less Or Equal?(x=w262, y=w334) -> (x <= y?=w387:bool)
    n125 = Or(x=w388, y=w387) -> (x .or. y?=w386:bool)
    n126 = Add(x=w355, y=w312) -> (x+y=w263:dbl)
    n127 = call "ObservadorPerturbacionPequeno.vi"("entrada planta"=w263, "salida planta"=w277, "xk +1"=w278) -> ("xk"=w279:T1)  [unwired: 7 in, 1 out]
    n128 = Multiply(x=w335, y=-1.0) -> (x*y=w337:dbl)
    n129 = Greater Or Equal?(x=w263, y=w335) -> (x >= y?=w390:bool)
    n130 = Less Or Equal?(x=w263, y=w337) -> (x <= y?=w389:bool)
    n131 = Greater Or Equal To 0?(x=w263) -> (x >= 0?=w339:bool)
    n132 = Less Than 0?(x=w263) -> (x < 0?=w338:bool)
    n133 = xnode "Digital output (1 sample) 3"("A/DIO2 (Pin 15)"=w339) -> ()  [unwired: 1 in, 1 out]
    n134 = xnode "Digital output (1 sample) 4"("A/DIO3 (Pin 17)"=w338) -> ()  [unwired: 1 in, 1 out]
    n135 = Or(x=w390, y=w389) -> (x .or. y?=w325:bool)
    n136 = case shown="True" w325 {
      tunnel: [w783 w784] -> w314
      tunnel: w263 -> [w782 _]
      frame False {
        n137 = Absolute Value(x=w782) -> (abs(x)=w783:dbl)
      }
      frame True {
        n138 = local read "saturacion"() -> (w784:dbl)
      }
    }
    n139 = shared-variable ".\\RT Variables.lvlib\\Homing"() -> (w371:bool)  [unwired: 1 in, 1 out]
    n140 = case shown="False" w386 {
      tunnel: [w779 w781] -> w365
      tunnel: w262 -> [w780 _]
      frame False {
        n141 = Absolute Value(x=w780) -> (abs(x)=w779:dbl)
      }
      frame True {
        n142 = local read "saturacion"() -> (w781:dbl)
      }
    }
    n143 = Select(t=T2."grande-Sensor" ("Enum"), s=w371, f=w367) -> (s? t:f=w323:T2)
    n144 = xnode "Analog input (1 sample)"() -> ("A/AI3 (Pin 9)"=w347:dbl)  [unwired: 1 in, 1 out]
    "sensor1" <- w347
    n145 = xnode "Analog input (1 sample) 2"() -> ("sensor2 (A/AI2 (Pin 7))"=w346:dbl)  [unwired: 1 in, 1 out]
    "sensor2 (A/AI2 (Pin 7))" <- w346
    n146 = Get Date/Time In Seconds() -> (seconds since 1Jan1904=w405:timestamp)
    n147 = Greater?(x=w347, y=3.0) -> (0:w366:bool)
    n148 = Greater?(x=w346, y=3.0) -> (0:w363:bool)
    n149 = case shown="\"grande-Sensor\"" w323 {
      tunnel: w314 -> [w479 _ _ _ _ _]
      tunnel: [w479 0.0 ("f") w492 0.3 ("f") w512 w526] -> w369
      tunnel: [T2."normal" ("Enum") w490 w501 w510 w518 w524] -> w368
      tunnel: w366 -> [_ w484 _ _ _ _]
      tunnel: w365 -> [w478 _ w498 _ _ _]
      tunnel: [w478 0.25 ("f") w498 0.0 ("f") w512 w526] -> w364
      tunnel: w363 -> [_ _ _ w502 _ _]
      tunnel: [_ _ w492 _ w517 _] -> w362
      tunnel: w361 -> [_ _ _ _ w516 _]
      tunnel: [_ w484 _ w506 _ _] -> w359
      tunnel: [_ w484 _ w506 _ w523] -> w357
      tunnel: [_ 1.0 _ _ _ _] -> w320
      tunnel: [_ TRUE _ w506 _ _] -> w321
      tunnel: w308 -> [_ _ w497 _ _ _]
      frame "normal", Default {
        n150 = local write "Numeric Control"(0.0) -> ()
      }
      frame "grande-Sensor" {
        # "Planta"
        n151 = Select(t=1.0, s=w484, f=0.0) -> (s? t:f=w481:dbl)
        n152 = local write "Numeric Control"(w481) -> ()
        n153 = shared-variable ".\\RT Variables.lvlib\\Homing"(FALSE) -> ()  [unwired: 1 in, 1 out]
        n154 = Select(t=T2."grande home" ("Enum"), s=w484, f=T2."grande-Sensor" ("Enum")) -> (s? t:f=w490:T2)
      }
      frame "grande home" {
        w492 = 0.0
        n155 = Absolute Value(x=w497) -> (abs(x)=w496:dbl)
        n156 = shared-variable ".\\RT Variables.lvlib\\Homing"(FALSE ("Homing")) -> ()  [unwired: 1 in, 1 out]
        n157 = Less?(x=w496, y=0.1) -> (x < y?=w494:bool)
        n158 = Select(t=T2."peque-sensor" ("Enum"), s=w494, f=T2."grande home" ("Enum")) -> (s? t:f=w501:T2)
      }
      frame "peque-sensor" {
        w506 = TRUE
        n159 = Select(t=-1.0, s=w502, f=0.0) -> (s? t:f=w503:dbl)
        n160 = local write "Numeric Control"(w503) -> ()
        n161 = Select(t=T2."peque- home" ("Enum"), s=w502, f=T2."peque-sensor" ("Enum")) -> (s? t:f=w510:T2)
      }
      frame "peque- home" {
        w512 = 0.0 ("f")
        n162 = shared-variable ".\\RT Variables.lvlib\\Set1 full"(1.0) -> ()  [unwired: 1 in, 1 out]
        n163 = Add(x=w516, y=1) -> (x+y=w517:dbl)
        n164 = Equal?(x=w517, y=100) -> (x = y?=w521:bool)
        n165 = Select(t=T2."peque-reset" ("Enum"), s=w521, f=T2."peque- home" ("Enum")) -> (s? t:f=w518:T2)
      }
      frame "peque-reset" {
        w523 = TRUE
        w526 = 0.0 ("f")
        n166 = Select(t=T2."normal" ("Enum"), s=w523, f=T2."peque-reset" ("Enum")) -> (s? t:f=w524:T2)
      }
    }
    n167 = local write "Reset Counter 2"(w357) -> ()
    n168 = local write "Reset Counter"(w359) -> ()
    n169 = Select(t=w320, s=w321, f=w262) -> (s? t:f=w322:dbl)
    n170 = xnode "Analog input (1 sample) 3"() -> ("stallBlanco (A/AI1 (Pin 5))"=w247:dbl, "stallRojo (A/AI0 (Pin 3))"=w249:dbl)  [unwired: 1 in, 1 out]
    "stallBlanco (A/AI1 (Pin 5))" <- w247
    "stallRojo (A/AI0 (Pin 3))" <- w249
    n171 = call <vilib>:"Set Duty Cycle.vi"("Duty Cycle"=w369, "PWM Ref In"=w370) -> ("error out"=w396:errorcluster, "PWM Ref Out"=w402:T4)  [unwired: 7 in]
    n172 = call <vilib>:"Set Duty Cycle.vi"("Duty Cycle"=w364, "PWM Ref In"=w398) -> ("error out"=w397:errorcluster, "PWM Ref Out"=w393:T4)  [unwired: 7 in]
    n173 = Multiply(x=0.987577800493881, y=w250) -> (x*y=w252:dbl)
    n174 = Multiply(x=0.012422199506119, y=w246) -> (x*y=w251:dbl)
    n175 = Multiply(x=0.987577800493881, y=w255) -> (x*y=w257:dbl)
    n176 = Multiply(x=0.012422199506119, y=w248) -> (x*y=w256:dbl)
    n177 = Add(x=w252, y=w251) -> (x+y=w244:dbl)
    n178 = Add(x=w257, y=w256) -> (x+y=w245:dbl)
    n179 = Bundle(w315, w245, "Counter Value"=w283, "seconds since 1Jan1904"=w405, w311, w244, "Counter Value"=w288) -> (w313:T26)  [unwired: 1 in]
    n180 = Merge Errors(w396, w397) -> (w395:errorcluster)
    n181 = shared-variable ".\\RT Variables.lvlib\\Stop RT Loops"() -> (w404:bool)  [unwired: 1 in, 1 out]
    n182 = Greater?(x=w245, y=0.1) -> (0:w374:bool)
    n183 = Greater?(x=w244, y=0.1) -> (0:w373:bool)
    n184 = xnode "Button"() -> ("Value"=w353:bool)  [unwired: 1 in, 1 out]
    n185 = shared-variable ".\\RT Variables.lvlib\\Data"(w313, error in=w395) -> (error out=w403:errorcluster)
    n186 = Or(x=w374, y=w373) -> (x .or. y?=w375:bool)
    n187 = Greater Or Equal To 0?(x=w322) -> (x >= 0?=w331:bool)
    n188 = Less Than 0?(x=w322) -> (x < 0?=w330:bool)
    n189 = Or(x=w403, y=w404) -> (x .or. y?=w392:bool)
    n190 = xnode "Digital output (1 sample)"("A/DIO0 (Pin 11)"=w331) -> ()  [unwired: 1 in, 1 out]
    n191 = Or(x=w353, y=w375) -> (x .or. y?=w372:bool)
    n192 = xnode "Digital output (1 sample) 2"("A/DIO1 (Pin 13)"=w330) -> ()  [unwired: 1 in, 1 out]
    n193 = Or(x=w392, y=w372) -> (x .or. y?=w391:bool)
  }
  n194 = Destroy Stream Endpoint(8:w61, 11:w60) -> (0:w58:errorcluster)
  n195 = node-c288(w64) -> ()  [unwired: 1 out]
  n196 = case shown="Error" w53 {
    selector: w53 -> [w822 w823]
    tunnel: [w822 w823] -> w15
    frame No Error {
      # "No action required."
    }
    frame Error {
      # "Destroys Message network stream to stop Message loop, in case of error."
      n197 = shared-variable ".\\RT Variables.lvlib\\2setpoint"() -> (w824:refnum<k21>)  [unwired: 1 in, 1 out]
      n198 = Destroy Stream Endpoint(11:w824) -> ()  [unwired: 1 in, 1 out]
    }
  }
  n199 = call <vilib>:"Stop.vi"("error in (no error)"=w15, "Encoder Ref In"=w45) -> ("error out"=w46:errorcluster, "Encoder Ref Out"=w47:T11)  [unwired: 8 in]
  n200 = call <vilib>:"Stop.vi"("error in (no error)"=w15, "Encoder Ref In"=w14) -> ("error out"=w17:errorcluster, "Encoder Ref Out"=w18:T11)  [unwired: 8 in]
  n201 = call <vilib>:"Close.vi"("error in (no error)"=w46, "Encoder Ref In"=w47) -> ("error out"=w40:errorcluster)  [unwired: 9 in]
  n202 = call <vilib>:"Close.vi"("error in (no error)"=w17, "Encoder Ref In"=w18) -> ("error out"=w16:errorcluster)  [unwired: 9 in]
  n203 = call <vilib>:"Close.vi"("error in (no error)"=w40, "PWM Ref In"=w37) -> ("error out"=w39:errorcluster)  [unwired: 9 in]
  n204 = call <vilib>:"Close.vi"("error in (no error)"=w16, "PWM Ref In"=w13) -> ("error out"=w12:errorcluster)  [unwired: 9 in]
  n205 = Merge Errors(w58, w57, w39, w12) -> (w56:errorcluster)
  n206 = shared-variable "myRIO-1900\\Network Shared Variables.lvlib\\error IO"(w56) -> ()  [unwired: 1 in, 1 out]
